vi "GetControlRefByArray.vi"(0 "VI Reference In":refnum<vi>, 7 "Control Path":string[](array[string]), 11 "error In":errorcluster) -> (4 "VI Reference Out":refnum<vi>, 8 "Ctl Refnum":refnum<vi>, 15 "error out":errorcluster)   [LabVIEW 2016]
doc: "<b>Gives the reference of controls in the input VI.</b>\n\nThe path of the control should be given in the successive index of the array"
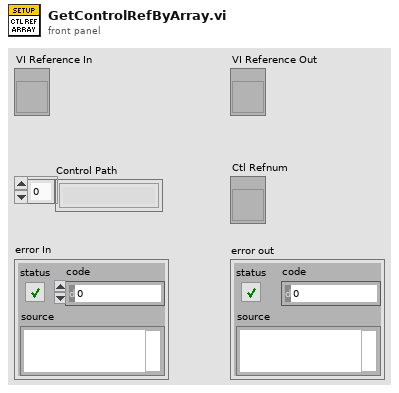
[diagram p1: front panel]
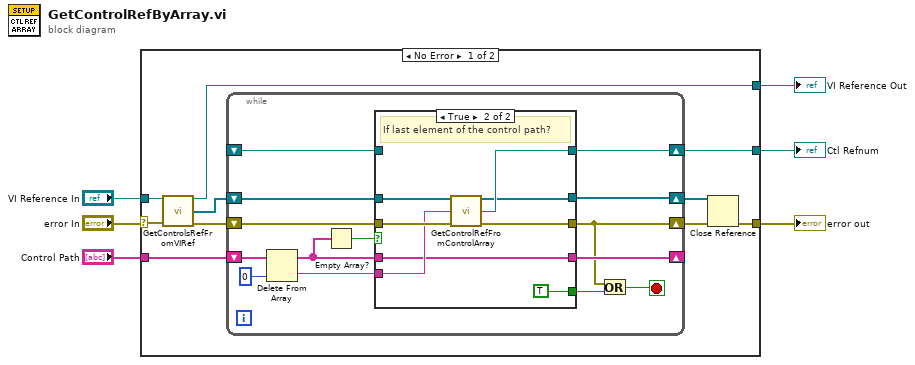
[diagram p0: block diagram]
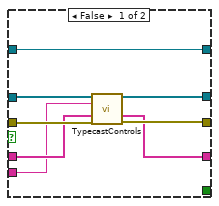
[diagram p2: hidden frame]
diagram:
  n1 = case shown="No Error" "error In" {
    selector: "error In" -> [w9 w48]
    tunnel: "Control Path" -> [w15 _]
    tunnel: [w8 w48] -> w5
    tunnel: [w12 _] -> w4
    tunnel: "VI Reference In" -> [w10 w47]
    tunnel: [w7 w47] -> w1
    frame No Error {
      n2 = call "GetControlsRefFromVIRef.vi"("VI Reference In"=w10, "Error In"=w9) -> ("VI Reference Out"=w7:refnum<vi>, "Controls[]"=w14:refnum<vi>[], "Error Out"=w11:errorcluster)  [unwired: 11 in]
      n3 = while {
        shift-right: [w18] -> w16
        shift-left: w11 -> [w28]
        shift-right: [w25] -> w13
        shift-left: w14 -> [w26]
        shift-right: [w21] -> w12
        shift-left: _ -> [w24]
        shift-right: [w23] -> _
        shift-left: w15 -> [w27]
        stop <- w17 stop-if-true
        n4 = Delete From Array(array=w27, index=0) -> (deleted portion=w29:string, array with subset deleted=w22:string[])  [unwired: 1 in]
        n5 = Empty Array?(array=w22) -> (empty?=w30:bool)
        n6 = case shown="True" w30 {
          tunnel: w26 -> [w38 w44]
          tunnel: w29 -> [w31 w45]
          tunnel: [w34 w42] -> w21
          tunnel: w28 -> [w37 w46]
          tunnel: [w35 w43] -> w18
          tunnel: [w36 w41] -> w25
          tunnel: w24 -> [w34 _]
          tunnel: [_ TRUE] -> w19
          tunnel: w22 -> [w33 w39]
          tunnel: [w32 w39] -> w23
          frame False {
            n7 = call "TypecastControls.vi"("Controls[]"=w38, "Control Name"=w31, "Control Path In"=w33, "error In"=w37) -> ("Sub Controls[]"=w36:refnum<vi>[], "Control Path Out"=w32:string[], "error out"=w35:errorcluster)  [unwired: 9 in]
          }
          frame True {
            # "If last element of the control path?"
            n8 = call "GetControlRefFromControlArray.vi"("Controls[]"=w44, "Control Name"=w45, "error In"=w46) -> ("Remaining Controls[]"=w41:refnum<vi>[], "Target Control"=w42:refnum<vi>, "error out"=w43:errorcluster)  [unwired: 10 in]
          }
        }
        n9 = Or(x=w18, y=w19) -> (x .or. y?=w17:bool)
      }
      n10 = Close Reference(reference=w13, error in (no error)=w16) -> (error out=w8:errorcluster)
    }
    frame Error {
    }
  }
  "Ctl Refnum" <- w4
  "error out" <- w5
  "VI Reference Out" <- w1
